vi "ReadFFLoop_thread.vi"(0 "board_sel":u32, 1 "exptus":u32=20000, 2 "ExtTrig":u8, 3 "btrig_ch":u8, 4 "blocktrigger":u8) -> ()   [LabVIEW 2015]
uses:
  ESLSCDLL.dll
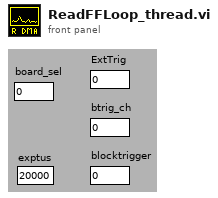
[diagram p1: front panel]
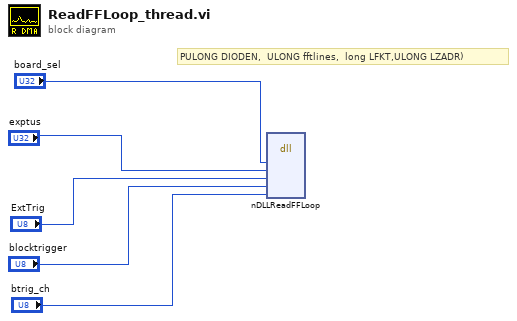
[diagram p0: block diagram]
diagram:
  # "PULONG DIODEN, \tULONG fftlines,  long LFKT,ULONG LZADR)"
  n1 = dll-call lib="C:/ENTW/PCIE/64bit/lv64/board.vis/ESLSCDLL.dll" fn="nDLLReadFFLoop" ("lwlscdll.dll:DLLReadFFLoop")("board_sel"="board_sel", "exptus"="exptus", "exttrig"="ExtTrig", "blocktrigger"="blocktrigger", "btrig_ch"="btrig_ch") -> ()  [unwired: 9 in, 2 out]
